vi "Parse Type.vi"(8 "error in (no error)":errorcluster, 9 "Text":string, 11 "ProtoParser in":refnum<class "ProtoParser.lvclass">) -> (0 "error out":errorcluster, 1 "Type":T1={"Type"=enum."double", "Subtype"=""}, 2 "Remaining":string, 3 "ProtoParser out":refnum<class "ProtoParser.lvclass">, 4 "Key Type":T1={"Type"=enum."double", "Subtype"=""}, 6 "Value Type":T1={"Type"=enum."double", "Subtype"=""})   [LabVIEW 2020, in "LV-Protoc.lvlib" / "ProtoParser.lvclass"]
doc: "Note, returns \"enum\" type for all unknown type names. \"enum\" types will need to be changed to \"message\" when warranted and validated separately."
uses:
  ProtoParser.lvclass
  LV-Proto/Type.ctl
  LV-Proto/Proto Type.ctl
  LV-Proto/LV-Proto.lvlib
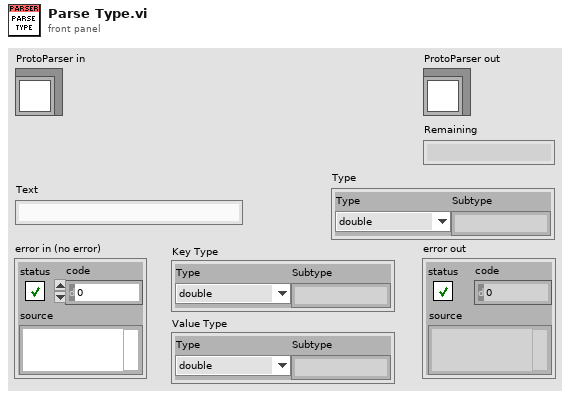
[diagram p1: front panel]
types:
  T1 = typedef "LV-Proto.lvlib/Type.ctl" = cluster{"Type":T2, "Subtype":string}
  T2 = typedef "LV-Proto.lvlib/Proto Type.ctl" = enum16{"UNKNOWN", "double", "float", "int32", "int64", "uint32", "uint64", "sint32", "sint64", "fixed32", "fixed64", "sfixed32", "sfixed64", "bool", "string", "bytes", "enum", "map", "message"}
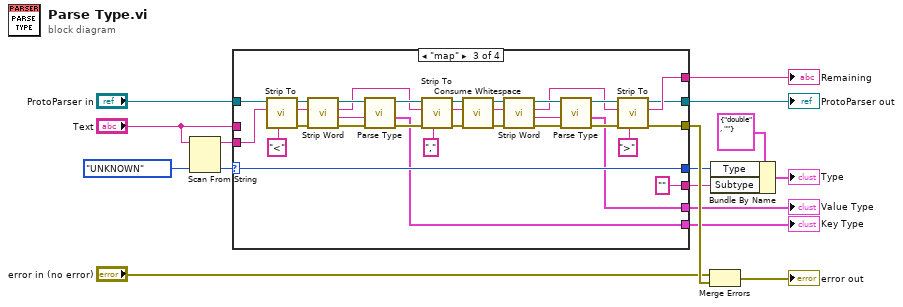
[diagram p0: block diagram]
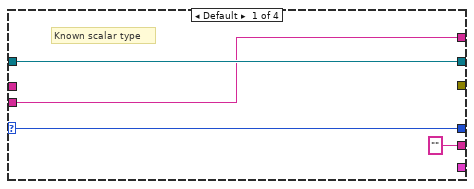
[diagram p2: hidden frame]
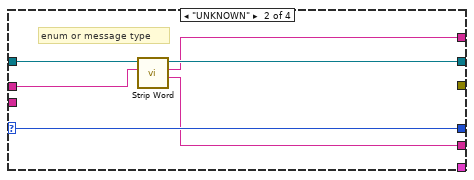
[diagram p3: hidden frame]
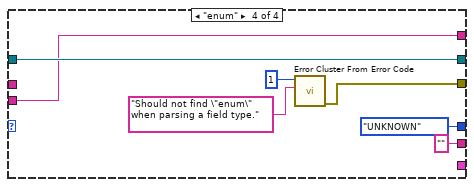
[diagram p4: hidden frame]
diagram:
  n1 = Scan From String(input string="Text", default 1=Proto_Type."UNKNOWN" ("Proto Type")) -> (remaining string=w13:string, output 1=w14:T2)  [unwired: 3 in, 2 out]
  n2 = case shown="\"map\"" w14 {
    selector: w14 -> [w19 w22 w56 _]
    tunnel: w13 -> [w18 _ w52 w64]
    tunnel: "Text" -> [_ w25 _ _]
    tunnel: "ProtoParser in" -> [w20 w26 w57 w65]
    tunnel: [w20 w24 w27 w65] -> w10
    tunnel: [w19 w22 w56 Proto_Type."UNKNOWN" ("Proto Type")] -> w5
    tunnel: [w18 w23 w28 w64] -> w9
    tunnel: ["" ("Word") w21 "" ("Word") "" ("Word")] -> w4
    tunnel: [_ _ w43 _] -> w3
    tunnel: [_ _ w30 _] -> w2
    tunnel: [_ _ w59 w66] -> w16
    frame Default {
      # "Known scalar type"
    }
    frame "UNKNOWN" {
      # "enum or message type"
      n3 = call "Strip Word.vi"("String"=w25, "ProtoParser in"=w26) -> ("Word"=w21:string, "Remaining"=w23:string, "ProtoParser out"=w24:refnum<class "ProtoParser.lvclass">)  [unwired: 6 in, 1 out]
    }
    frame "map" {
      n4 = call "Strip To.vi"("End"="<", "String"=w52, "ProtoParser in"=w57) -> ("error out"=w46:errorcluster, "Remaining"=w51:string, "ProtoParser out"=w54:refnum<class "ProtoParser.lvclass">)  [unwired: 5 in, 1 out]
      n5 = call "Strip Word.vi"("error in (no error)"=w46, "String"=w51, "ProtoParser in"=w54) -> ("error out"=w45:errorcluster, "Word"=w50:string, "Remaining"=w39:string, "ProtoParser out"=w49:refnum<class "ProtoParser.lvclass">)  [unwired: 5 in]
      n6 = call "Parse Type.vi"("error in (no error)"=w45, "Text"=w50, "ProtoParser in"=w49) -> ("error out"=w44:errorcluster, "Type"=w43:T1, "ProtoParser out"=w47:refnum<class "ProtoParser.lvclass">)  [unwired: 3 in, 3 out]
      n7 = call "Strip To.vi"("End"=",", "error in (no error)"=w44, "String"=w39, "ProtoParser in"=w47) -> ("error out"=w40:errorcluster, "Remaining"=w41:string, "ProtoParser out"=w42:refnum<class "ProtoParser.lvclass">)  [unwired: 4 in, 1 out]
      n8 = call "Consume Whitespace.vi"("error in (no error)"=w40, "String"=w41, "ProtoParser in"=w42) -> ("error out"=w34:errorcluster, "Remaining"=w35:string, "ProtoParser out"=w36:refnum<class "ProtoParser.lvclass">)  [unwired: 6 in]
      n9 = call "Strip Word.vi"("error in (no error)"=w34, "String"=w35, "ProtoParser in"=w36) -> ("error out"=w38:errorcluster, "Word"=w37:string, "Remaining"=w31:string, "ProtoParser out"=w33:refnum<class "ProtoParser.lvclass">)  [unwired: 5 in]
      n10 = call "Parse Type.vi"("error in (no error)"=w38, "Text"=w37, "ProtoParser in"=w33) -> ("error out"=w58:errorcluster, "Type"=w30:T1, "ProtoParser out"=w32:refnum<class "ProtoParser.lvclass">)  [unwired: 3 in, 3 out]
      n11 = call "Strip To.vi"("End"=">", "error in (no error)"=w58, "String"=w31, "ProtoParser in"=w32) -> ("error out"=w59:errorcluster, "Remaining"=w28:string, "ProtoParser out"=w27:refnum<class "ProtoParser.lvclass">)  [unwired: 4 in, 1 out]
    }
    frame "enum" {
      n12 = call <vilib>:"Error Cluster From Error Code.vi"("error message (\"\")"="Should not find \"enum\" when parsing a field type.", "error code (0)"=1) -> ("error out"=w66:errorcluster)  [unwired: 7 in]
    }
  }
  "ProtoParser out" <- w10
  "Remaining" <- w9
  "Key Type" <- w3
  "Value Type" <- w2
  n13 = Merge Errors("error in (no error)", w16) -> (→"error out":errorcluster)
  n14 = Bundle By Name(cluster=T1 {"Type"=enum."double", "Subtype"=""} ("Subtype"), "Type"=w5, "Subtype"=w4) -> (→"Type":T1)
